vi "Tool_Unicode Update Listbox Data.vi"(5 "Interpret as Unicode (T)":bool=TRUE, 6 "error in (no error)":errorcluster, 8 "Data[]":string[](array[string]), 9 "Listbox Ref":refnum<vi>) -> (0 "error out":errorcluster, 3 "Listbox Ref":refnum<vi>)   [LabVIEW 2009]
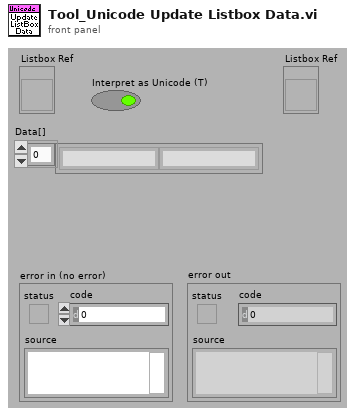
[diagram p1: front panel]
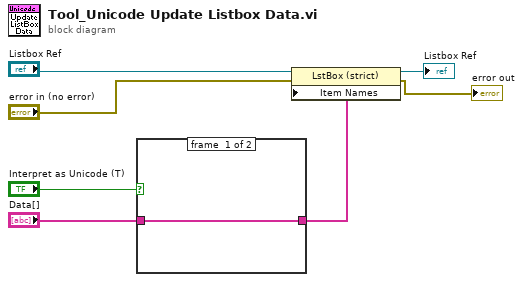
[diagram p0: block diagram]
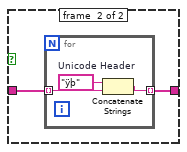
[diagram p2: hidden frame]
diagram:
  n1 = case shown="True" "Interpret as Unicode (T)" {
    tunnel: "Data[]" -> [w8 w10]
    tunnel: [w8 w9] -> w1
    frame #0 {
    }
    frame #1 {
      n2 = for {
        tunnel: w10 -> [w13] mode=indexing
        tunnel: [w12] -> w9 mode=indexing
        w11 = "ÿþ"  # Unicode Header
        n3 = Concatenate Strings(w11, w13) -> (w12:string)
      }
    }
  }
  n4 = property class="LstBox (strict)"(reference="Listbox Ref", error in="error in (no error)", "Item Names"=w1) -> (reference out=→"Listbox Ref":refnum<vi>, error out=→"error out":errorcluster)
